vi "2DGaussianRotationModelwithOffset.vi"(3 "output control":T1, 4 "data":T2, 5 "X":dbl[](array[numeric]), 6 "a":dbl[](array[numeric])) -> (0 "error out":errorcluster, 1 "f'(X,a)":dbl[][](array[numeric]), 2 "f(X,a)":dbl[](array[numeric]))   [LabVIEW 2012]
doc: "This template is the starting point for creating a model function to be passed to the Nonlinear Curve Fit.vi."
uses:
  <vilib>/gmath/NumericalOptimization/objective function data.ctl
  <vilib>/gmath/NumericalOptimization/LM_output select.ctl
  <vilib>/Analysis/Matrix/Numeric/Conversions/Array To Matrix - RA2.vi
  <vilib>/Analysis/baseanly.llb/A x Vector.vi
  <vilib>/Analysis/NI_AALBase.lvlib
  <vilib>/Analysis/Matrix/NI_Matrix.lvlib
  <vilib>/gmath/NI_Gmath.lvlib
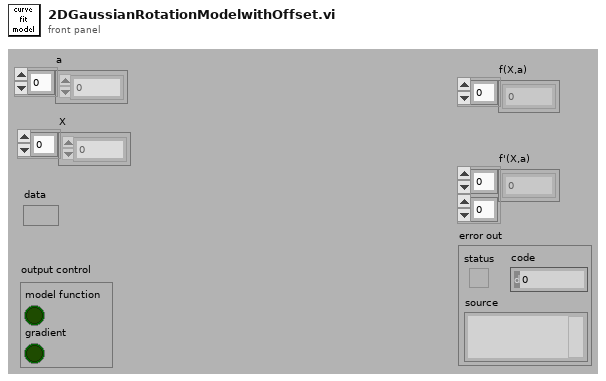
[diagram p1: front panel]
types:
  T1 = typedef "NI_Gmath.lvlib/LM_output select.ctl" = cluster{"model function":bool, "gradient":bool}
  T2 = typedef "NI_Gmath.lvlib/objective function data.ctl" = variant
  T3 = typedef "NI_Matrix.lvlib/RealMatrix.ctl" = dbl[][]
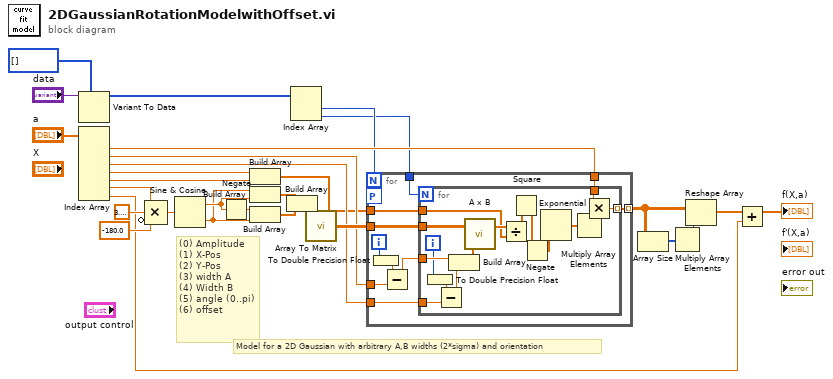
[diagram p0: block diagram]
diagram:
  # "Model for a 2D Gaussian with arbitrary A,B widths (2*sigma) and orientation"
  # "(0) Amplitude\n(1) X-Pos\n(2) Y-Pos\n(3) width A\n(4) Width B\n(5) angle (0..pi)\n(6) offset"
  n1 = Variant To Data(type=i32[] [], Variant="data") -> (data=w3:i32[])  [unwired: 1 in, 1 out]
  n2 = Index Array(array="a") -> (element #1=w19:dbl, element #2=w13:dbl, element #3=w12:dbl, element #4=w18:dbl, element #5=w17:dbl, element #6=w11:dbl, element #7=w5:dbl)  [unwired: 7 in]
  n3 = Compound Arithmetic op=MULTIPLY(w11, 3.141592653589793, invert -180.0 ("value")) -> (w10:dbl)
  n4 = Sine & Cosine(0:w10) -> (1:w28:dbl, 2:w27:dbl)
  n5 = Negate(x=w28) -> (-x=w29:dbl)
  n6 = Build Array(w18, w17) -> (w7:dbl[])
  n7 = Build Array(w27, w28) -> (w26:dbl[])
  n8 = Build Array(w29, w27) -> (w25:dbl[])
  n9 = Build Array(w26, w25) -> (w24:dbl[][])
  n10 = Index Array(array=w3) -> (element #1=w2:i32, element #2=w1:i32)  [unwired: 2 in]
  n11 = call-poly <vilib>:"Array To Matrix.vi"("Real 2D Array"=w24) -> ("Real Matrix"=w23:T3)
  n12 = for {
    N: w2 -> [_]
    tunnel: w23 -> [w39]
    tunnel: w7 -> [w38]
    tunnel: [w37] -> w22 mode=indexing
    tunnel: w19 -> [w36]
    tunnel: w1 -> [w35]
    tunnel: w13 -> [w32]
    tunnel: w12 -> [w30]
    workers-P: _ -> [_]
    i -> [w34]
    n13 = To Double Precision Float(number=w34) -> (double precision float=w33:dbl)
    n14 = Subtract(x=w33, y=w32) -> (x-y=w31:dbl)
    n15 = for {
      N: w35 -> [_]
      tunnel: w31 -> [w55]
      tunnel: w39 -> [w53]
      tunnel: w38 -> [w51]
      tunnel: [w48] -> w37 mode=indexing
      tunnel: w36 -> [w47]
      tunnel: w30 -> [w44]
      i -> [w46]
      n16 = To Double Precision Float(number=w46) -> (double precision float=w45:dbl)
      n17 = Subtract(x=w45, y=w44) -> (x-y=w43:dbl)
      n18 = Build Array(w55, w43) -> (w54:dbl[])
      n19 = call-poly <vilib>:"A x B.vi"("Vector"=w54, "A"=w53) -> ("A x Vector"=w52:dbl[])  [unwired: 1 out]
      n20 = Divide(x=w52, y=w51) -> (x/y=w42:dbl[])
      n21 = Square(x=w42) -> (x^2=w41:dbl[])
      n22 = Negate(x=w41) -> (-x=w40:dbl[])
      n23 = Exponential(1:w40) -> (0:w50:dbl[])
      n24 = Multiply Array Elements(1:w50) -> (0:w49:dbl)
      n25 = Multiply(x=w47, y=w49) -> (x*y=w48:dbl)
    }
  }
  n26 = Array Size(array=w22) -> (size(s)=w20:i32[])
  n27 = Multiply Array Elements(1:w20) -> (0:w21:i32)
  n28 = Reshape Array(w22, w21) -> (w14:dbl[])
  n29 = Add(x=w14, y=w5) -> (x+y=→"f(X,a)":dbl[])
